vi "Create_PDF4Box_stats.vi"(0 "Tableau de valves":string[](array[string])=["112105740008010001", "112105740008010002", "112105740008010003", "112105740008010004", "112105740008010005", "112105740008010006", "112105740008010007", "112105740008010008", "112105740008010009", "112105740008010010", "112105740008010011", "112105740008010012", "112105740008010013", "112105740008010014", "112105740008010015", "112105740008010016", "112105740008010017", "112105740008010018", "112105740008010019", "112105740008010020", "112105740008010021", "112105740008010022", "112105740008010023", "112105740008010024", "112105740008010025"], 1 "Produit":string="12-216C-04521 EQIFIL 417mA 14.4ohm", 2 "Client":string="EMS Electro Medical System", 3 "Nombre Cartons":string="4", 4 "Numero Carton":string="1", 5 "Cust_Prod_Ref":string="EL-360", 6 "Cust_Indice":string="03", 7 "error in (no error)":errorcluster caption="entrée d'erreur (pas d'erreur)", 8 "Commande":string="03838/08-01.07.01", 9 "Cust_Order":string="CF-08-0253/2") -> (27 "error out":errorcluster caption="sortie d'erreur")   [LabVIEW 2020]
doc: "Le fichier modèle (BoxFile.txt) pour le générateur de PDF doit se trouver dans le répertoire:\n\\data\\pydist\nLe PDF généré pour le carton se trouve aussi dans ce répertoire après sa création\nL'executable python pour la génération du PDF se trouve dans ce même répertoire,\nl'appel de ce générateur se fait avec la ligne de commande : \n\\data\\pydist\\Create_Cust_PDF4Box.exe\nPour l'instrant l'éxécutable Python ne gère qu'1 feuille PDF pouvant contenir au maximum\n40 codes barre, à modifier si nécessaire (pas plus de 25/box selon CDC...)"
uses:
  <vilib>/Utility/NIReport.llb/NI_ReportGenerationCore.lvlib
panel:
  out "standard output (Batch)":string caption="sortie standard"
  out "standard error (Batch)":string caption="erreur standard"
  out "return code (Batch)":i32 caption="code de retour"
  out "default printer":string caption="imprimante par défaut"
  out "system configured printers":string[](array[string]) caption="imprimantes système configurées"
  in  "Nom de l'executable":string="Create_Cust_PDF4Box.exe"
  # "FONCTIONNEMENT OK :\nVoir les commentaires du script\n\"PDF2printer.bat\" pour explications.\nEn cas de changement du fonctionnement,\non peut agir directement avec ce script sur\ncertains paramêtres."
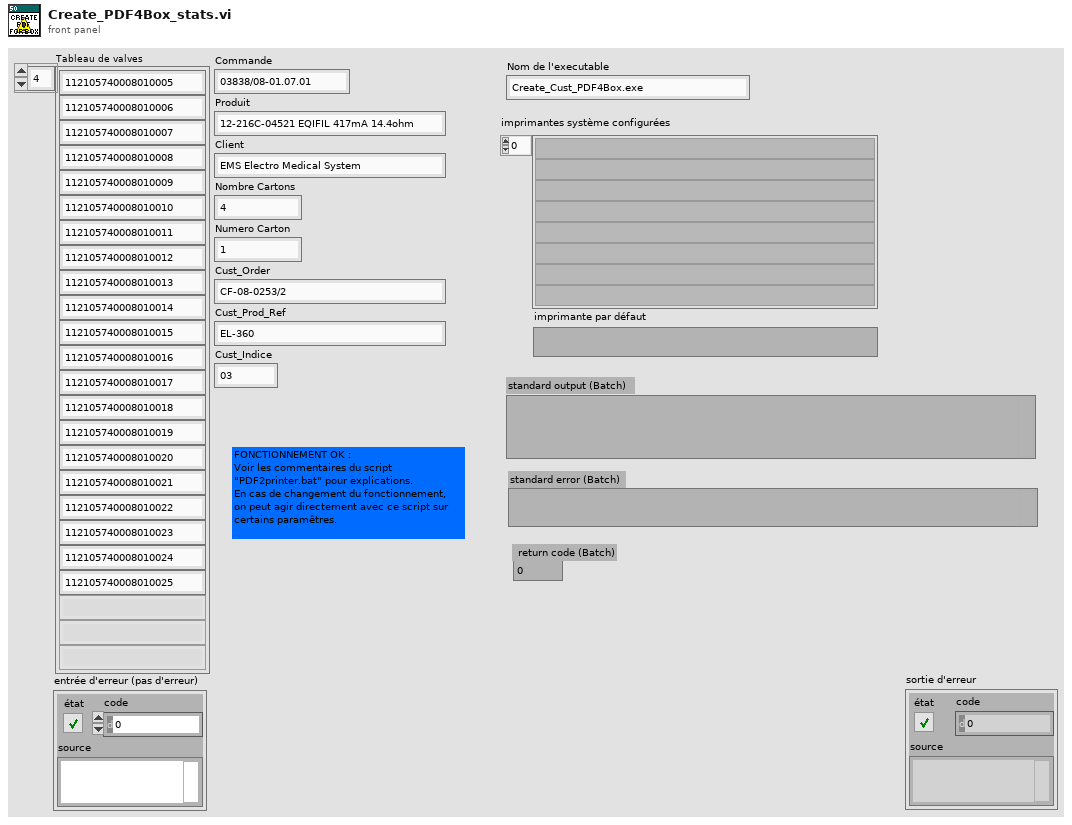
[diagram p1: front panel]
types:
  T1 = enum16{"open", "replace", "create", "open or create", "replace or create", "replace or create with confirmation"}
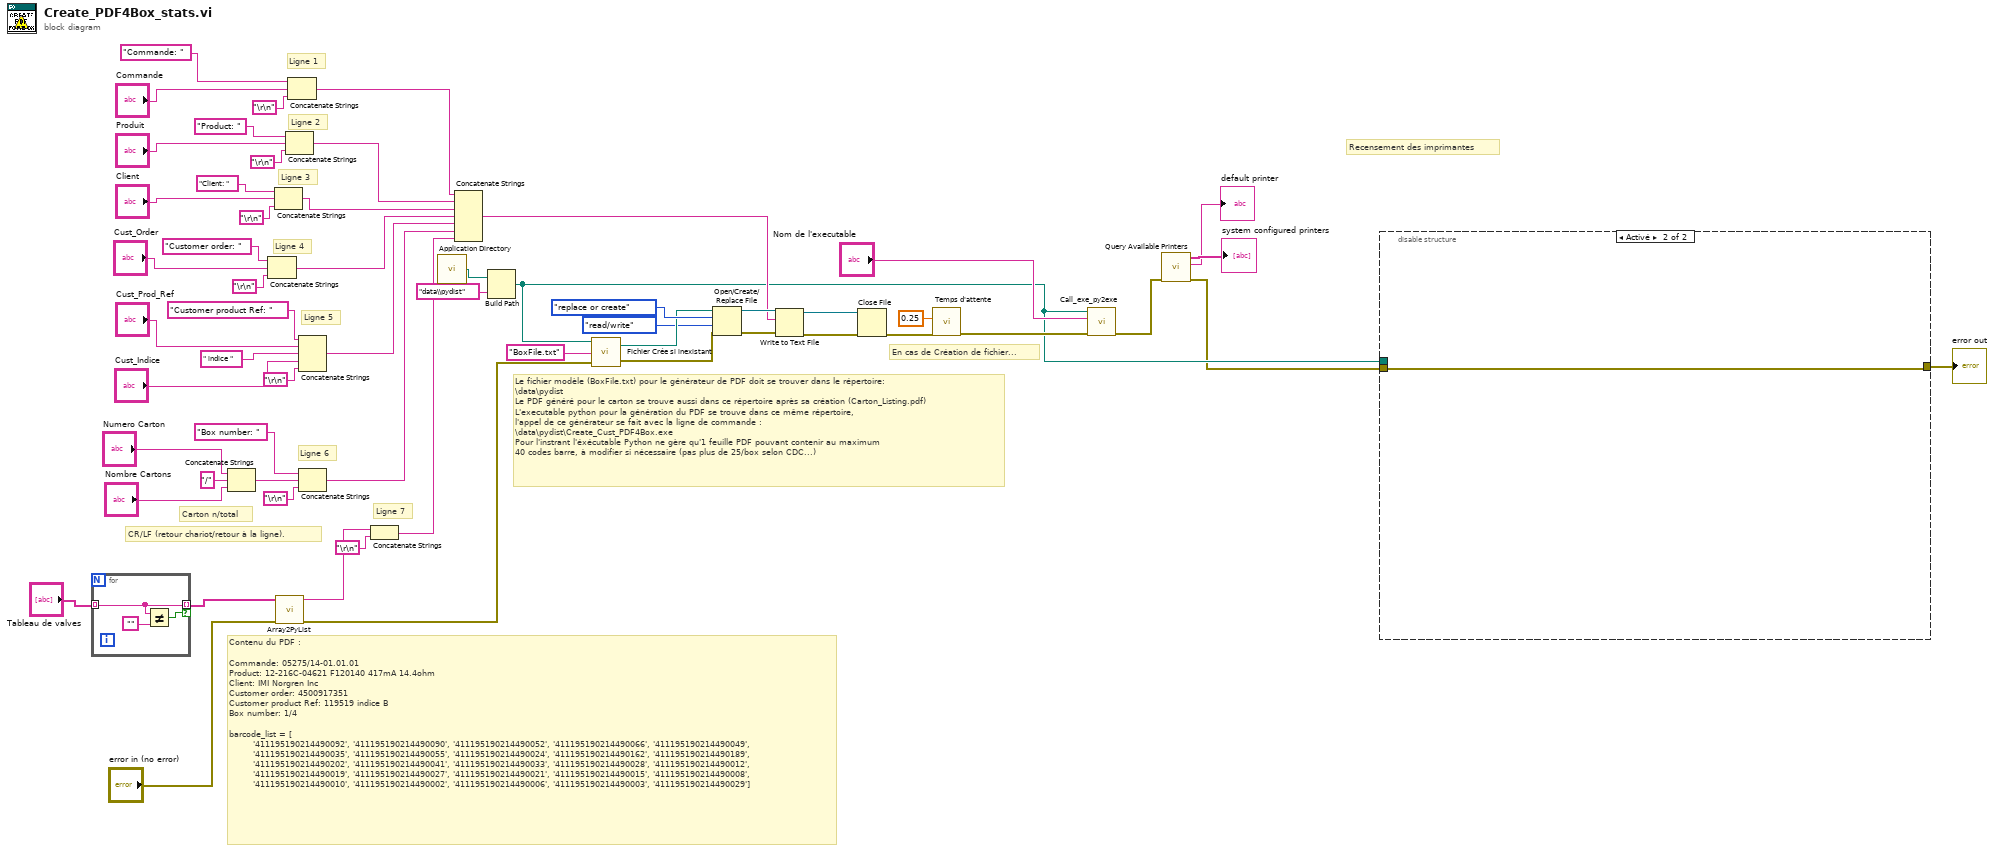
[diagram p0: block diagram]
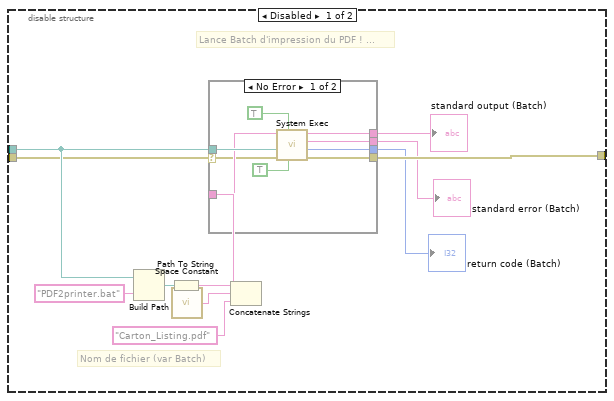
[diagram p2: hidden frame]
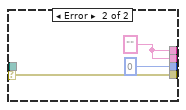
[diagram p3: hidden frame]
diagram:
  # "Recensement des imprimantes"
  # "En cas de Création de fichier..."
  # "Le fichier modèle (BoxFile.txt) pour le générateur de PDF doit se trouver dans le répertoire:\n\\data\\pydist\nLe PDF généré pour le carton se trouve aussi dans ce répertoire après sa création (Carton_Listing.pdf)\nL'executable python pour la génération du PDF se trouve dans ce même répertoire,\nl'appel de ce générateur se fait avec la ligne de commande : \n\\data\\pydist\\Create_Cust_PDF4Box.exe\nPour l'instrant l'éxécutable Python ne gère qu'1 feuille PDF pouvant contenir au maximum\n40 codes barre, à modifier si nécessaire (pas plus de 25/box selon CDC...)"
  # "Ligne 7"
  # "Ligne 6"
  # "Ligne 5"
  # "Ligne 4"
  # "Ligne 3"
  # "Ligne 2"
  # "Ligne 1"
  # "CR/LF (retour chariot/retour à la ligne)."
  # "Carton n/total"
  # "Contenu du PDF : \n\nCommande: 05275/14-01.01.01\nProduct: 12-216C-04621 F120140 417mA 14.4ohm\nClient: IMI Norgren Inc\nCustomer order: 4500917351\nCustomer product Ref: 119519 indice B\nBox number: 1/4\n\nbarcode_list = [\n        '411195190214490092', '411195190214490090', '411195190214490052', '411195190214490066', '411195190214490049',\n        '411195190214490035', '411195190214490055', '411195190214490024', '411195190214490162', '411195190214490189',\n        '411195190214490202', '411195190214490041', '411195190214490033', '411195190214490028', '411195190214490012',\n        '411195190214490019', '411195190214490027', '411195190214490021', '411195190214490015', '411195190214490008',\n        '411195190214490010', '411195190214490002', '411195190214490006', '411195190214490003', '411195190214490029']"
  n1 = for {
    tunnel: "Tableau de valves" -> [w61] mode=indexing
    tunnel: [w61] -> w1 mode=indexing if=w60
    n2 = Not Equal?(x=w61, y="") -> (x != y?=w60:bool)
  }
  n3 = Concatenate Strings("Numero Carton", "/", "Nombre Cartons") -> (w53:string)
  n4 = Concatenate Strings("Customer order: ", "Cust_Order", "\r\n") -> (w22:string)
  n5 = Concatenate Strings("Client: ", "Client", "\r\n") -> (w23:string)
  n6 = call "Array2PyList.vi"("error in (no error)"="error in (no error)", "Tableau de valves"=w1) -> ("error out"=w26:errorcluster, "List_Valves"=w32:string)  [unwired: 8 in]
  n7 = Concatenate Strings("Product: ", "Produit", "\r\n") -> (w24:string)
  n8 = Concatenate Strings("Commande: ", "Commande", "\r\n") -> (w25:string)
  n9 = Concatenate Strings("Customer product Ref: ", "Cust_Prod_Ref", " indice ", "Cust_Indice", "\r\n") -> (w21:string)
  n10 = Concatenate Strings("Box number: ", w53, "\r\n") -> (w20:string)
  n11 = Concatenate Strings(w32, "\r\n") -> (w19:string)
  n12 = call <vilib>:"Application Directory.vi"() -> ("Application Directory"=w13:path)
  n13 = Concatenate Strings(w25, w24, w23, w22, w21, w20, w19) -> (w18:string)
  n14 = Build Path(base path=w13, name or relative path="data\\pydist" ("nom ou chemin relatif")) -> (appended path=w5:path)
  n15 = call "Fichier Crée si inexistant.vi"("error in"=w26, "nom fichier"="BoxFile.txt", "chemin du dossier IN"=w5) -> ("error out"=w17:errorcluster, "chemin sous dossier OUT"=w31:path)
  n16 = Open/Create/Replace File(file path (use dialog)=w31, error in=w17, operation (0:open)=T1."replace or create" ("opération (0 : open)"), access (0:read/write)=enum16{"read/write", "read-only", "write-only"}."read/write" ("accès (0 : read/write)")) -> (refnum out=w30:refnum<file>, error out=w29:errorcluster)  [unwired: 2 in, 1 out]
  n17 = Write to Text File(file (use dialog)=w30, text=w18, error in=w29) -> (refnum out=w27:refnum<file>, error out=w28:errorcluster)  [unwired: 1 in, 1 out]
  n18 = Close File(refnum=w27, error in=w28) -> (error out=w10:errorcluster)  [unwired: 1 out]
  n19 = call "Temps d'attente"("error in (no error)"=w10, "Delay Time (s)"=0.25) -> ("error out"=w9:errorcluster)  [unwired: 9 in]
  n20 = call "Call_exe_py2exe.vi"("error in (no error)"=w9, "Nom de l'executable"="Nom de l'executable", "Répertoire de travail"=w5) -> ("error out"=w6:errorcluster)  [unwired: 8 in]
  n21 = call <vilib>:"Query Available Printers.vi"("error in (no error)"=w6) -> ("error out"=w3:errorcluster, "default printer"=→"default printer":string, "system configured printers"=→"system configured printers":string[])  [unwired: 8 in]
  n22 = disable-structure shown="Activé" {
    disable-tunnel: w5 -> [w70 _]
    disable-tunnel: [w66 w86] -> w4
    disable-tunnel: w3 -> [w62 w86]
    frame Disabled {
      # "Nom de fichier (var Batch)"
      # "Lance Batch d'impression du PDF ! ..."
      n23 = Build Path(base path=w70, name or relative path="PDF2printer.bat" ("nom ou chemin relatif")) -> (appended path=w72:path)
      n24 = Path To String(path=w72) -> (string=w71:string)
      n25 = call <vilib>:"Space Constant.vi"() -> ("String"=w68:string)
      n26 = Concatenate Strings(w71, w68, "Carton_Listing.pdf" ("nom fichier")) -> (w69:string)
      n27 = case shown="No Error" w62 {
        selector: w62 -> [w74 w85]
        tunnel: w70 -> [w81 _]
        tunnel: w69 -> [w80 _]
        tunnel: [w79 w85] -> w66
        tunnel: [w78 0 ("return code")] -> w65
        tunnel: [w77 w83] -> w64
        tunnel: [w76 w83] -> w63
        frame No Error {
          n28 = call <vilib>:"System Exec.vi"("run minimized? (F)"=TRUE, "wait until completion? (T)"=TRUE, "error in (no error)"=w74, "working directory"=w81, "command line"=w80) -> ("error out"=w79:errorcluster, "return code"=w78:i32, "standard error"=w77:string, "standard output"=w76:string)  [unwired: 3 in]
        }
        frame Error {
          w83 = "" ("standard error")
        }
      }
      "return code (Batch)" <- w65
      "standard error (Batch)" <- w64
      "standard output (Batch)" <- w63
    }
    frame Enabled {
    }
  }
  "error out" <- w4
